vi "OpenSystemDefinitionFile.vi"(8 "error in (no error)":errorcluster, 11 "VeriStand Test Case in":refnum<class "VeriStandTestCase.lvclass">) -> (0 "error out":errorcluster, 3 "VeriStand Test Case out":refnum<class "VeriStandTestCase.lvclass">)   [LabVIEW 2016, in "VeriStandTestCase.lvclass"]
uses:
  VeriStandTestCase.lvclass
  VeriStandTestCase.lvclass/VeriStandTestCase.ctl
  <vilib>/NI VeriStand/Execution/Workspace/NI_VS Workspace ExecutionAPI.lvlib
  VeriStandTestUtilities/VeriStandTestUtilities.lvlib
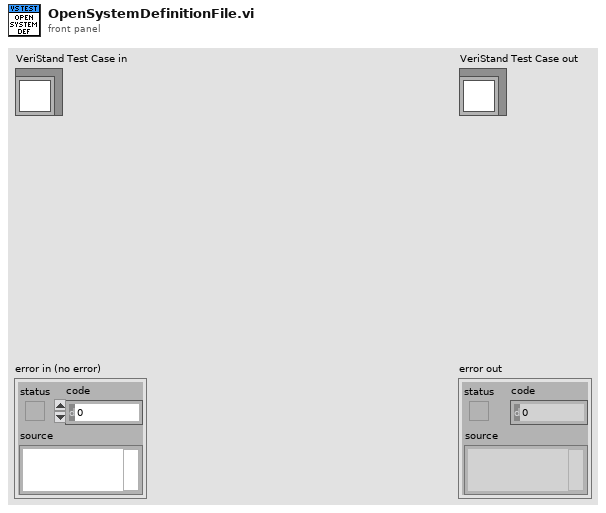
[diagram p1: front panel]
types:
  T1 = typedef "NI_VS Workspace ExecutionAPI.lvlib/WorkspaceAPI.ctl" = refnum<k24>
  T2 = typedef "VeriStandTestUtilities.lvlib/SystemDefinitionInformation.ctl" = cluster{"Path":path, "Target Information List":T3[]}
  T3 = typedef "VeriStandTestUtilities.lvlib/TargetInformation.ctl" = cluster{"Name":string, "IP Address":string, "Operating System":string, "Target Rate":dbl, "Chassis List":T4[], "Custom Device List":string[]}
  T4 = typedef "VeriStandTestUtilities.lvlib/ChassisInformation.ctl" = cluster{"Name":string, "Devices":string[]}
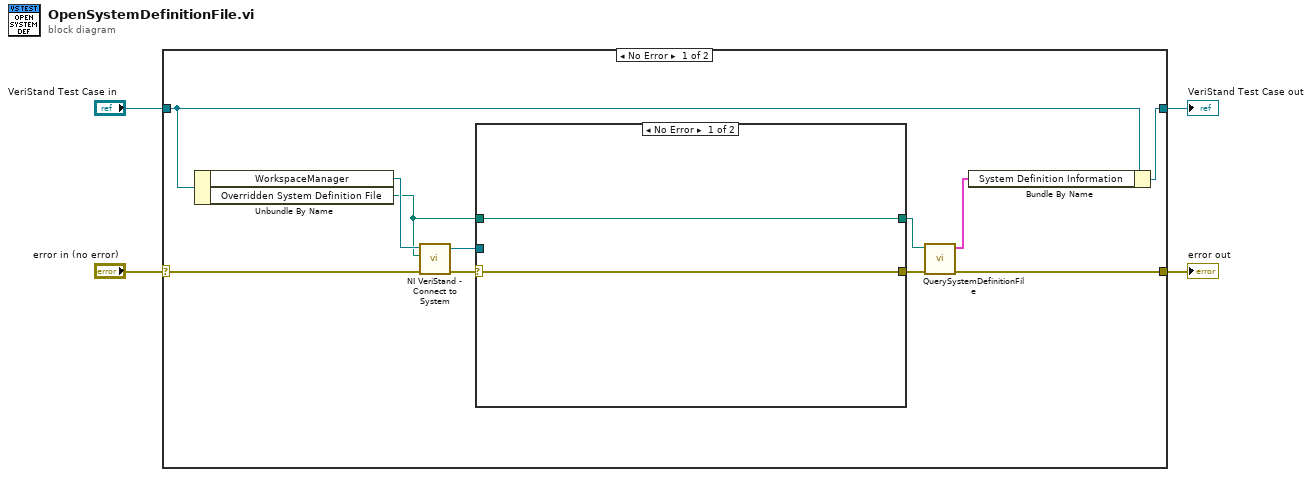
[diagram p0: block diagram]
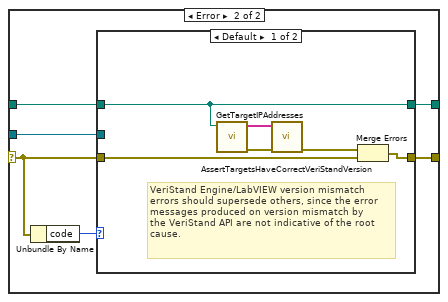
[diagram p2: hidden frame]
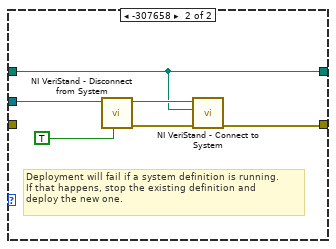
[diagram p3: hidden frame]
diagram:
  n1 = case shown="No Error" "error in (no error)" {
    selector: "error in (no error)" -> [w13 w37]
    tunnel: [w8 w37] -> w4
    tunnel: [w9 w36] -> w2
    tunnel: "VeriStand Test Case in" -> [w10 w36]
    frame No Error {
      n2 = Unbundle By Name(w10) -> ("WorkspaceManager"=w14:T1, "Overridden System Definition File"=w5:path)
      n3 = call <vilib>:"NI VeriStand - Connect to System.vi"("error in (no error)"=w13, "System Definition File (.nivssdf)"=w5, "WorkspaceManager in"=w14) -> ("error out"=w12:errorcluster, "WorkspaceManager out"=w11:T1)  [unwired: 7 in]
      n4 = case shown="No Error" w12 {
        selector: w12 -> [w17 w20]
        tunnel: [w17 w23] -> w15
        tunnel: w5 -> [w16 w22]
        tunnel: w11 -> [_ w21]
        tunnel: [w16 w18] -> w7
        frame No Error {
        }
        frame Error {
          n5 = Unbundle By Name(w20) -> ("code"=w19:i32)
          n6 = case shown="Default" w19 {
            tunnel: w20 -> [w27 _]
            tunnel: [w29 w35] -> w23
            tunnel: w21 -> [_ w33]
            tunnel: w22 -> [w24 w30]
            tunnel: [w24 w30] -> w18
            frame Default {
              # "VeriStand Engine/LabVIEW version mismatch\nerrors should supersede others, since the error\nmessages produced on version mismatch by\nthe VeriStand API are not indicative of the root\ncause."
              n7 = call "GetTargetIPAddresses.vi"("absolute system definition file"=w24) -> ("error out"=w25:errorcluster, "ip addresses"=w26:string[])  [unwired: 9 in]
              n8 = call "AssertTargetsHaveCorrectVeriStandVersion.vi"("error in (no error)"=w25, "targets"=w26) -> ("error out"=w28:errorcluster)  [unwired: 9 in]
              n9 = Merge Errors(w28, w27) -> (w29:errorcluster)
            }
            frame -307658 {
              # "Deployment will fail if a system definition is running.\nIf that happens, stop the existing definition and\ndeploy the new one."
              n10 = call <vilib>:"NI VeriStand - Disconnect from System.vi"("Undeploy System Definition (F)"=TRUE, "WorkspaceManager in"=w33) -> ("error out"=w34:errorcluster, "WorkspaceManager out"=w32:T1)  [unwired: 8 in]
              n11 = call <vilib>:"NI VeriStand - Connect to System.vi"("error in (no error)"=w34, "System Definition File (.nivssdf)"=w30, "WorkspaceManager in"=w32) -> ("error out"=w35:errorcluster)  [unwired: 7 in, 1 out]
            }
          }
        }
      }
      n12 = call "QuerySystemDefinitionFile.vi"("error in (no error)"=w15, "System Definiton File in"=w7) -> ("error out"=w8:errorcluster, "System Definition Information out"=w6:T2)  [unwired: 8 in]
      n13 = Bundle By Name(cluster=w10, "System Definition Information"=w6) -> (w9:refnum<class "VeriStandTestCase.lvclass">)
    }
    frame Error {
    }
  }
  "error out" <- w4
  "VeriStand Test Case out" <- w2
